vi "Get_Logging_Data.vi"(8 "error in (no error)":errorcluster, 11 ".NET Reference in":refnum<k24>) -> (0 "error out":errorcluster, 1 "data out":dbl[](array[numeric]), 2 "datapoint":i32, 3 "Reference out":refnum<k24>)   [LabVIEW 2017]
uses:
  D:/test/FULLband-sts/Fullband_Sample/DLL/InstrumentDLL.dll
  DLL/InstrumentDLL.dll
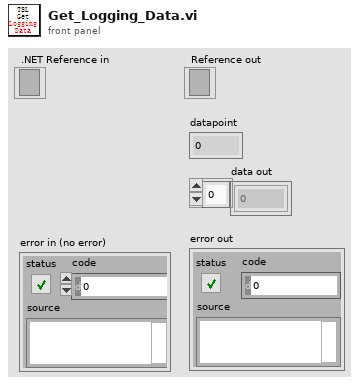
[diagram p1: front panel]
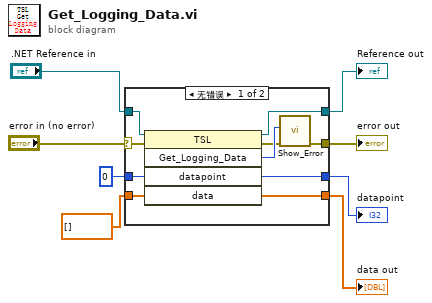
[diagram p0: block diagram]
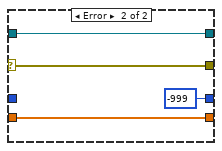
[diagram p2: hidden frame]
diagram:
  n1 = case shown="无错误" "error in (no error)" {
    selector: "error in (no error)" -> [w9 w22]
    tunnel: [w18 w19] -> w8
    tunnel: ".NET Reference in" -> [w17 w21]
    tunnel: [w16 w21] -> w6
    tunnel: [w10 w22] -> w5
    tunnel: [w15 -999 ("datapoint")] -> w4
    tunnel: dbl[] [] ("data") -> [w14 w19]
    tunnel: 0 ("datapoint") -> [w13 _]
    frame No Error {
      n2 = invoke on="调用节点" class="TSL" method="Get_Logging_Data"(reference=w17, error in=w9, "datapoint"=w13, "data"=w14) -> (reference out=w16:refnum<k24>, error out=w11:errorcluster, "Get_Logging_Data"=w12:i32, "datapoint"=w15:i32, "data"=w18:dbl[])  [unwired: 1 in]
      n3 = call "Show_Error.vi"("error in (no error)"=w11, "Error"=w12) -> ("error out"=w10:errorcluster)  [unwired: 9 in]
    }
    frame Error {
    }
  }
  "data out" <- w8
  "Reference out" <- w6
  "error out" <- w5
  "datapoint" <- w4
